vi "TestVI.vi"() -> ()   [LabVIEW 2012]
panel:
  in  "working directory":path=path "C:/Users/eol-lidar-admin/WVD-MCSupdate/tempShare/NetCDFexplorations/TestScriptsPython_Perl"
  in  "command line":string="C:\\Users\\eol-lidar-admin\\AppData\\Local\\Programs\\Python\\Python36-32\\python.exe C:\\Users\\eol-lidar-admin\\WVD-MCSupdate\\tempShare\\NetCDFexplorations\\TestScriptsPython_Perl\\MyScript.py thing1 thing2"
  out "error out":errorcluster
  out "standard error":string
  out "standard output":string="This is a test python script\r\nThese are the arguments I passed in to my test script:\r\nthing1\r\nthing2\r\n"
  # "This command will run this in a new process"
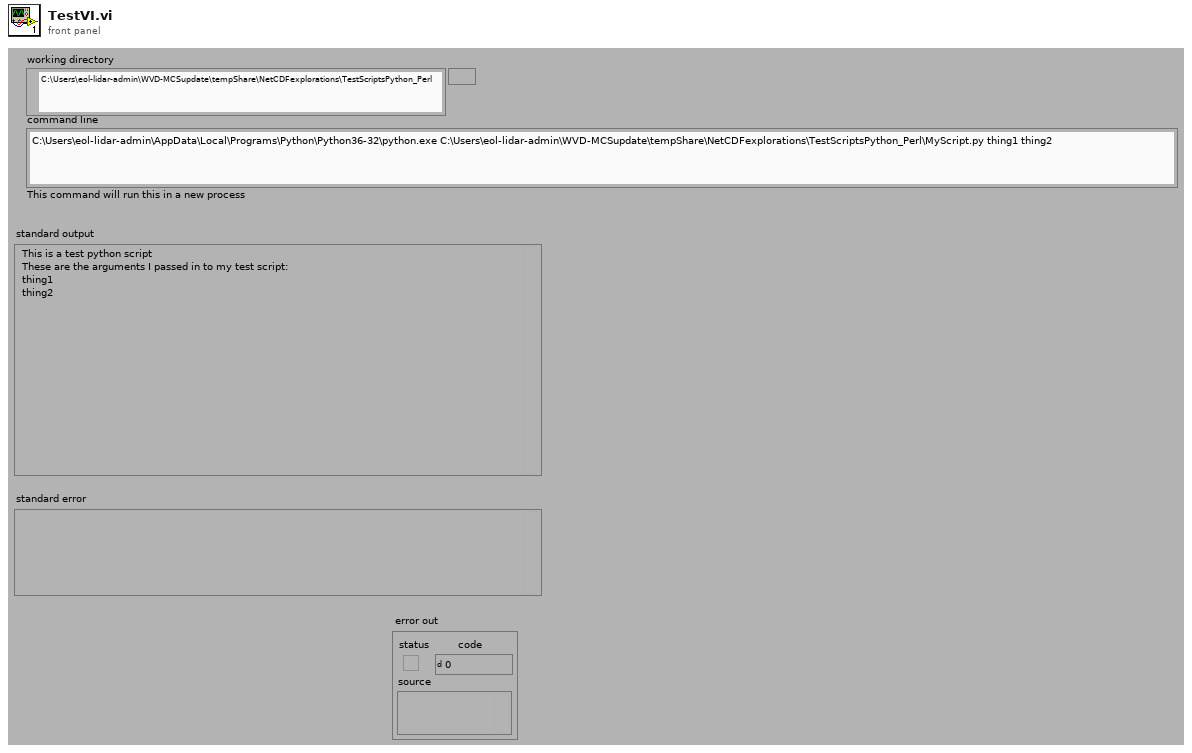
[diagram p1: front panel]
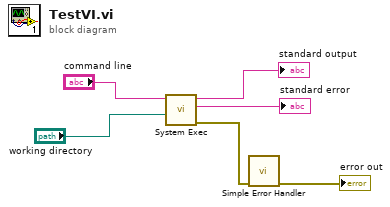
[diagram p0: block diagram]
diagram:
  n1 = call <vilib>:"System Exec.vi"("working directory"="working directory", "command line"="command line") -> ("error out"=w2:errorcluster, "standard error"=→"standard error":string, "standard output"=→"standard output":string)  [unwired: 4 in, 3 out]
  n2 = call <vilib>:"Simple Error Handler.vi"("error in (no error)"=w2) -> ("error out"=→"error out":errorcluster)  [unwired: 1 in, 7 out]
